vi "Temp-1.vi"() -> ()   [LabVIEW 2022 SP3]
panel:
  out "Anzahl Regelungen":dbl
  out "Zeit":string
  out "Datum":string
  out "Kurvenverläufe":T1(graph)
  out "Kühlung ein":bool
  out "Heizung ein":bool
  out "Untere Temperatur [°C]":dbl
  out "Obere Temperatur [°C]":dbl
  in  "Hysterese [°C]":dbl
  in  "Temperatur [°C]":dbl
  in  "stop (F)":bool caption="Stopp (F)"
  # "Temperaturregelung"
  # "Eingabewerte"
  # "Grenzwerte"
  # "Aktuelle Werte [°C]"
  # "Temperatur"
  # "maximal Temp."
  # "minimal Temp."
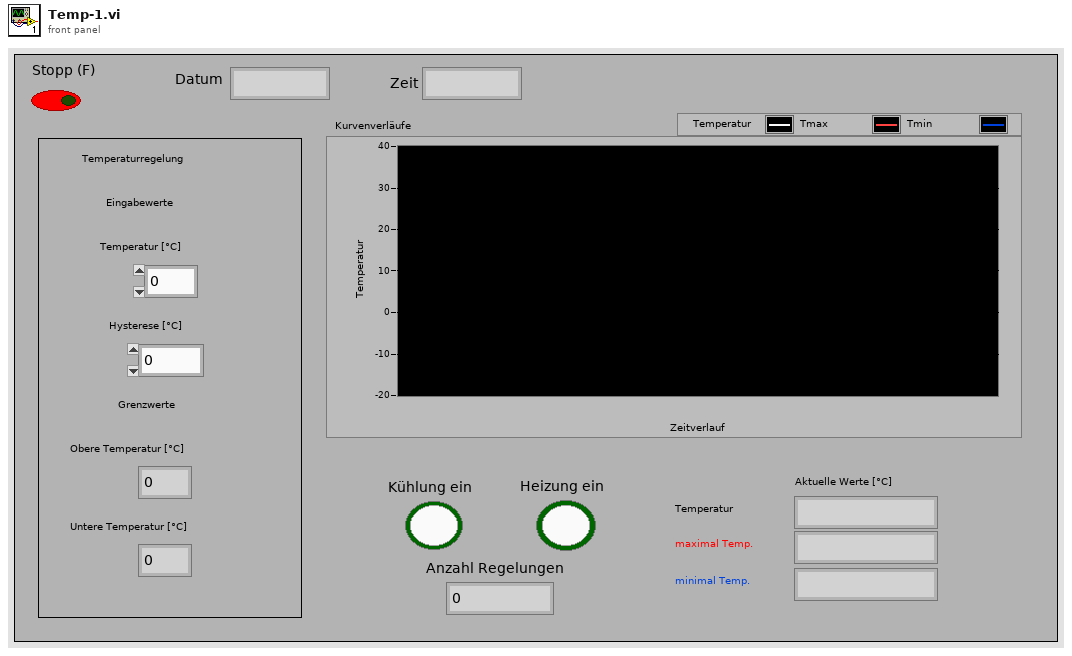
[diagram p1: front panel]
types:
  T1 = cluster{"Zufalszahl":dbl, "Zufalszahl":dbl, "Zufalszahl":dbl}
  T2 = cluster{"Zufalszahl":dbl, "Zufalszahl":dbl, "Zufalszahl":dbl}[]
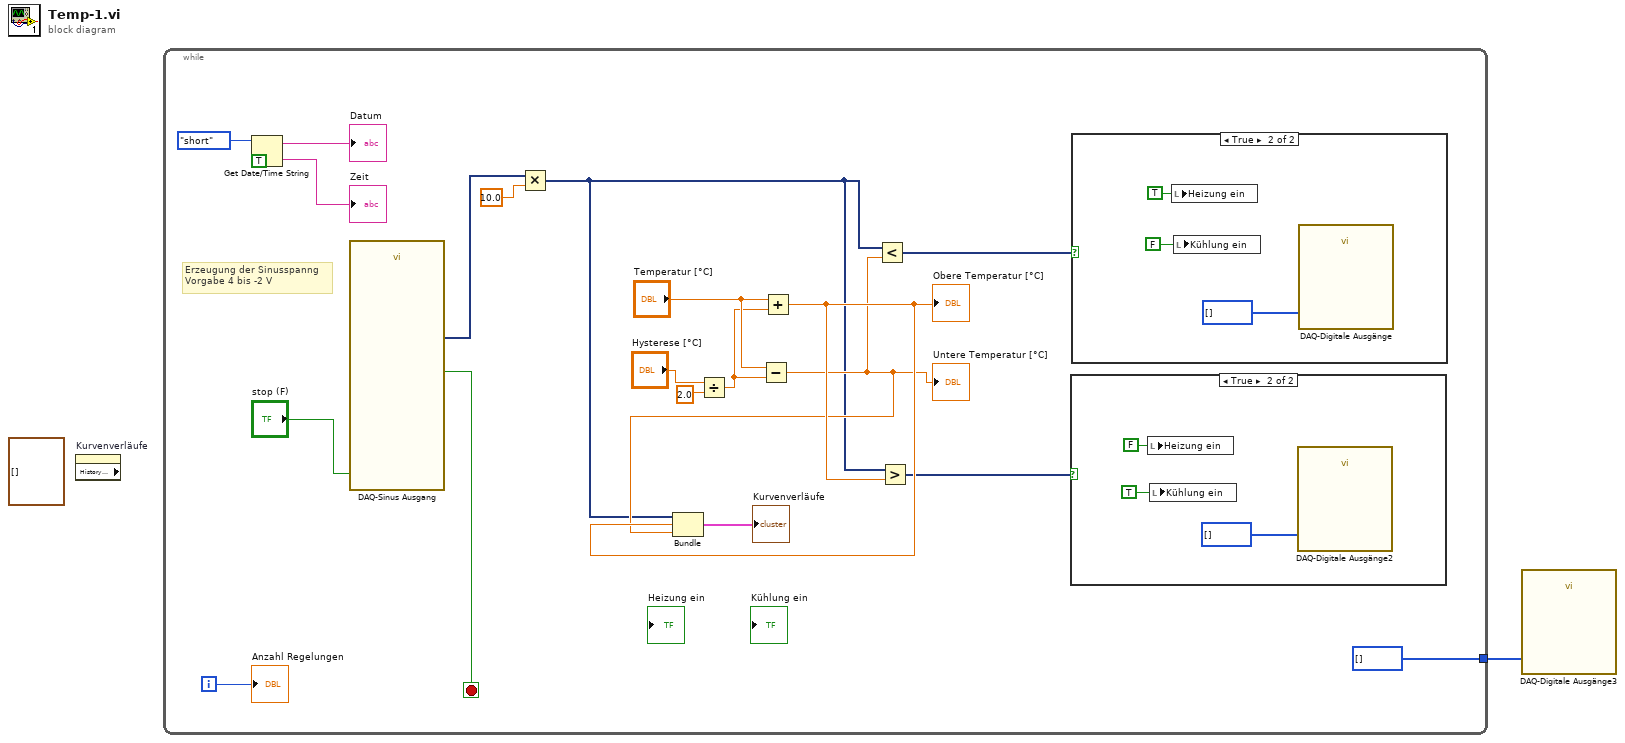
[diagram p0: block diagram]
diagram:
  (unwired) T2 [] ("Historiendaten")
  n1 = property on="Kurvenverläufe" class="WFChart (strict)" props=["History Data"]() -> ()  [unwired: 2 in, 3 out]
  n2 = while {
    tunnel: [u32[] [] ("data")] -> w1
    i -> [w8]
    stop <- w20 stop-if-true
    # "Erzeugung der Sinusspanng\nVorgabe 4 bis -2 V"
    n3 = Get Date/Time String(date format (0)=enum16{"short", "long", "abbreviated"}."short" ("Datumsformat (0)"), want seconds? (F)=TRUE ("Angabe von Sekunden? (F)")) -> (date string=→"Datum":string, time string=→"Zeit":string)  [unwired: 1 in]
    n4 = call "DAQ-Sinus Ausgang"("stop (F)"="stop (F)") -> ("data"=w17:dynamicdata, "stopped"=w20:bool)  [unwired: 15 in, 2 out]
    n5 = Multiply(x=w17, y=10.0) -> (x*y=w13:dynamicdata)
    n6 = Divide(x="Hysterese [°C]", y=2.0) -> (x/y=w5:dbl)
    n7 = Subtract(x="Temperatur [°C]", y=w5) -> (x-y=w15:dbl)
    "Untere Temperatur [°C]" <- w15
    n8 = Add(x="Temperatur [°C]", y=w5) -> (x+y=w16:dbl)
    "Obere Temperatur [°C]" <- w16
    n9 = Bundle ("Bündeln")(w13, w16, w15) -> (→"Kurvenverläufe":cluster{dynamicdata, dbl, dbl})  [unwired: 1 in]
    n10 = Less?(x=w13, y=w15) -> (x < y?=w4:dynamicdata)
    n11 = Greater?(x=w13, y=w16) -> (0:w3:dynamicdata)
    n12 = case shown="True" w3 {
      frame False {
      }
      frame True {
        n13 = local write "Heizung ein"(FALSE ("Heizung ein")) -> ()
        n14 = local write "Kühlung ein"(TRUE ("Kühlung ein 2")) -> ()
        n15 = call "DAQ-Digitale Ausgänge2"("data"=u32[] []) -> ()  [unwired: 17 in, 2 out]
      }
    }
    n16 = case shown="True" w4 {
      frame False {
      }
      frame True {
        n17 = local write "Heizung ein"(TRUE ("Heizung ein")) -> ()
        n18 = local write "Kühlung ein"(FALSE ("Kühlung ein 2")) -> ()
        n19 = call "DAQ-Digitale Ausgänge"("data"=u32[] []) -> ()  [unwired: 17 in, 2 out]
      }
    }
    "Anzahl Regelungen" <- w8
  }
  n20 = call "DAQ-Digitale Ausgänge3"("data"=w1) -> ()  [unwired: 17 in, 2 out]
